vi "GV-DrawYaxisLscale.vi"(5 "Dir":bool, 6 "Picture IN":picture, 7 "Stacked?":bool, 8 "error in (no error)":errorcluster, 10 "Plot":i32, 11 "Gviewer in":refnum<class "Gviewer.lvclass">) -> (0 "error out":errorcluster, 3 "Gviewer out":refnum<class "Gviewer.lvclass">, 4 "Picture OUT":picture)   [LabVIEW 2020, in "Sgraph_lib_V1.lvlib" / "Gviewer.lvclass"]
doc: "Draw an Y-scale on the graph canvas"
uses:
  Gviewer.lvclass
  Gviewer.lvclass/Gviewer.ctl
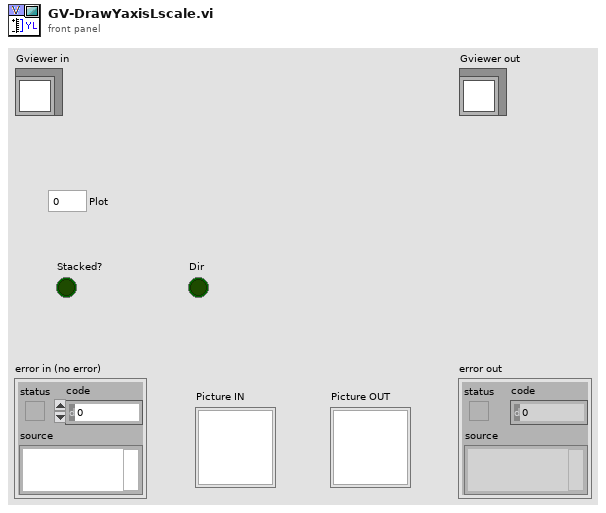
[diagram p1: front panel]
types:
  T1 = cluster{"coordinate 1":i16, "value 1":dbl, "coordinate 2":i16, "value 2":dbl, "log?(F)":bool}
  T2 = cluster{"horizontal":bool, "left/top":bool, "draw bar":bool, "line color":u32, "text color(black)":u32}
  T3 = cluster{"data":dbl[], "max":dbl[], "min":dbl[], "Status":u32[]}[]
  T4 = typedef "Sgraph_lib_V1.lvlib/Gviewer.lvclass/Typedef_SelProperties.ctl" = cluster{"Color":u32, "LineType":T5, "max":dbl, "min":dbl, "unit":string}
  T5 = typedef "Sgraph_lib_V1.lvlib/Gviewer.lvclass/Typedef_LineType.ctl" = enum16{"num_bare", "num_MinMax_Area", "num_MinMax_Lines", "num_MinMax_Forfor", "num_Max_Area", "num_Max_Line", "num_Max_Forfor", "num_Min_Area", "num_Min_Line", "num_Min_Fosfor", "Boolean_Line_01", "Boolean_Area_01", "Boolean_Fosfor_01", "Boolean_Line_TF", "Boolean_Area_TF", "Boolean_Fosfor_TF", "Boolean_OnOff_Line", "Boolean_OnOff_Area", "Boolean_OnOff_Fosfor", "Boolean_spare", "StringEvent_Line", "StringEvent_TimeLine"}
  T6 = cluster{"data":dbl[], "max":dbl[], "min":dbl[], "Status":u32[]}
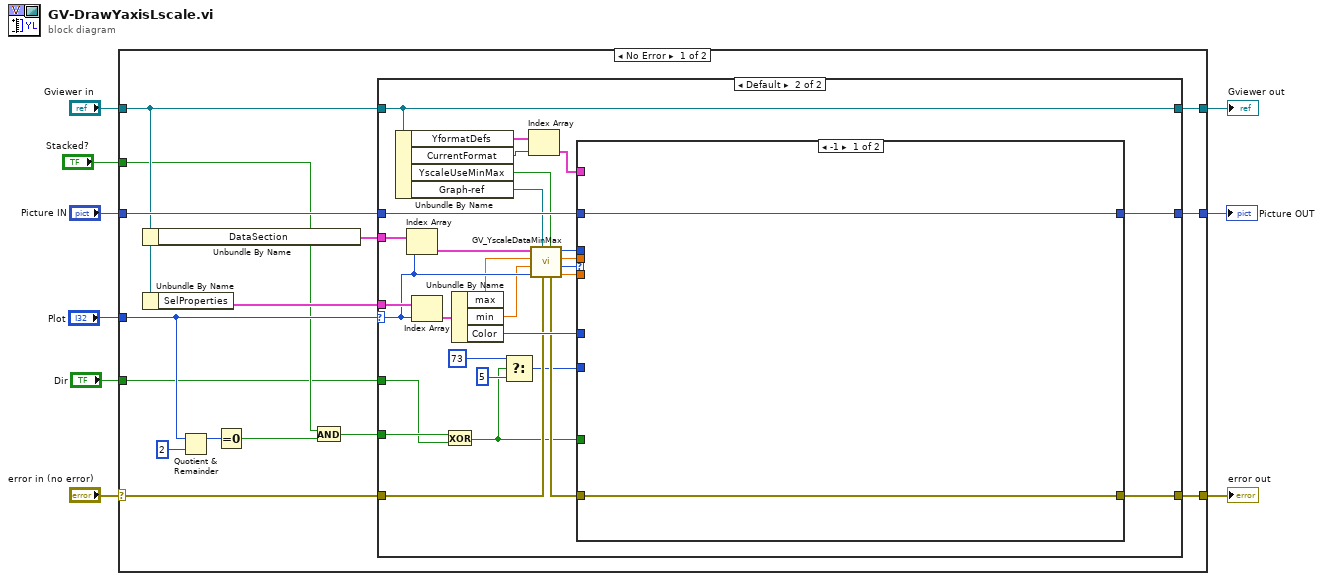
[diagram p0: block diagram]
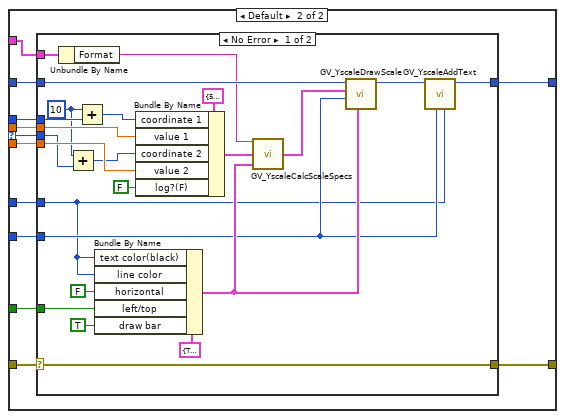
[diagram p3: hidden frame]
diagram:
  n1 = case shown="No Error" "error in (no error)" {
    selector: "error in (no error)" -> [w19 w99]
    tunnel: [w18 w99] -> w8
    tunnel: [w17 w98] -> w6
    tunnel: "Gviewer in" -> [w20 w98]
    tunnel: "Picture IN" -> [w23 w97]
    tunnel: [w24 w97] -> w4
    tunnel: "Plot" -> [w16 _]
    tunnel: "Stacked?" -> [w13 _]
    tunnel: "Dir" -> [w10 _]
    frame No Error {
      n2 = Unbundle By Name(w20) -> ("DataSection"=w21:T3)
      n3 = Unbundle By Name(w20) -> ("SelProperties"=w22:T4[])
      n4 = Quotient & Remainder(x=w16, y=2) -> (x-y*floor(x/y)=w14:i32)  [unwired: 1 out]
      n5 = Equal To 0?(x=w14) -> (x = 0?=w12:bool)
      n6 = And(x=w13, y=w12) -> (x .and. y?=w11:bool)
      n7 = case shown="Default" w16 {
        selector: w16 -> [_ w47]
        tunnel: [w26 w56] -> w24
        tunnel: w23 -> [w26 w55]
        tunnel: w22 -> [_ w54]
        tunnel: w21 -> [_ w51]
        tunnel: w20 -> [w27 w43]
        tunnel: w19 -> [w25 w46]
        tunnel: [w25 w41] -> w18
        tunnel: [w27 w43] -> w17
        tunnel: w11 -> [_ w30]
        tunnel: w10 -> [_ w29]
        frame -1 {
        }
        frame Default {
          n8 = Unbundle By Name(w43) -> ("YformatDefs"=w38:cluster{"Description":string, "Format":string}[], "CurrentFormat"=w37:i32, "YscaleUseMinMax"=w34:bool, "Graph-ref"=w35:refnum<vi>)
          n9 = Index Array(array=w51, index=w47) -> (element=w50:T6)
          n10 = Index Array(array=w54, index=w47) -> (element=w53:T4)
          n11 = Exclusive Or(1:w29, 2:w30) -> (0:w28:bool)
          n12 = Unbundle By Name(w53) -> ("max"=w40:dbl, "min"=w39:dbl, "Color"=w52:u32)
          n13 = Select(t=73 ("y"), s=w28, f=5 ("y")) -> (s? t:f=w31:i32)
          n14 = Index Array(array=w38, index=w37) -> (element=w36:cluster{"Description":string, "Format":string})
          n15 = call "GV_YscaleDataMinMax.vi"("IncludeMinMax"=w34, "error in (no error)"=w46, "Graph-ref"=w35, "Plot"=w47, "Scale-min"=w39, "Scale-max"=w40, "PAQ-data"=w50) -> ("min"=w48:dbl, "Coord-min"=w44:i32, "max"=w49:dbl, "Coord-max"=w45:i32, "error out"=w42:errorcluster)
          n16 = case shown="-1" w44 {
            selector: w44 -> [_ w63]
            tunnel: [w58 w70] -> w56
            tunnel: w55 -> [w58 w69]
            tunnel: w31 -> [_ w68]
            tunnel: w52 -> [_ w67]
            tunnel: w49 -> [_ w66]
            tunnel: w48 -> [_ w65]
            tunnel: w45 -> [_ w64]
            tunnel: w42 -> [w57 w62]
            tunnel: [w57 w61] -> w41
            tunnel: w36 -> [_ w60]
            tunnel: w28 -> [_ w59]
            frame -1 {
            }
            frame Default {
              n17 = case shown="No Error" w62 {
                selector: w62 -> [w79 w96]
                tunnel: [w92 w95] -> w70
                tunnel: w69 -> [w91 w95]
                tunnel: w68 -> [w88 _]
                tunnel: w67 -> [w85 _]
                tunnel: w66 -> [w81 _]
                tunnel: w65 -> [w80 _]
                tunnel: w64 -> [w75 _]
                tunnel: w63 -> [w74 _]
                tunnel: [w79 w96] -> w61
                tunnel: w60 -> [w78 _]
                tunnel: w59 -> [w71 _]
                frame No Error {
                  w73 = 10 ("x")
                  n18 = Unbundle By Name(w78) -> ("Format"=w77:string)
                  n19 = Add(x=w73, y=w74) -> (x+y=w72:i32)
                  n20 = Add(x=w73, y=w75) -> (x+y=w76:i32)
                  n21 = Bundle By Name(cluster=T2 {"horizontal"=TRUE, "left/top"=FALSE, "draw bar"=FALSE, "line color"=0, "text color(black)"=0} ("scale attributes"), "text color(black)"=w85, "line color"=w85, "horizontal"=FALSE, "left/top"=w71, "draw bar"=TRUE) -> (w89:T2)
                  n22 = Bundle By Name(cluster=T1 {"coordinate 1"=5, "value 1"=5.0, "coordinate 2"=5, "value 2"=5.0, "log?(F)"=FALSE} ("scale definition"), "coordinate 1"=w76, "value 1"=w81, "coordinate 2"=w72, "value 2"=w80, "log?(F)"=FALSE) -> (w83:T1)
                  n23 = call "GV_YscaleCalcScaleSpecs.vi"("FormatString"=w77, "scale definition"=w83, "scale attributes"=w89) -> ("scale specs"=w94:cluster{"coordinate":i16, "label":string}[])  [unwired: 6 in]
                  n24 = call "GV_YscaleDrawScale.vi"("scale attributes"=w89, "constant coordinate"=w88, "scale specs"=w94, "picture"=w91) -> ("new picture"=w93:picture)  [unwired: 7 in]
                  n25 = call "GV_YscaleAddText.vi"("Color"=w85, "X-position"=w88, "2D Picture IN"=w93) -> ("2D Picture OUT"=w92:picture)  [unwired: 8 in]
                }
                frame Error {
                }
              }
            }
          }
        }
      }
    }
    frame Error {
    }
  }
  "error out" <- w8
  "Gviewer out" <- w6
  "Picture OUT" <- w4
